vi "setUp.vi"(8 "error in (no error)":errorcluster, 11 "reference in":refnum<class "test.lvclass">) -> (0 "error out":errorcluster, 3 "reference in":refnum<class "test.lvclass">)   [LabVIEW 2011, in "test.lvclass"]
doc: "setUp runs prior to the test method during test execution. Use this method to initialize any object data required by your tests."
uses:
  test.lvclass
  test.lvclass/test.ctl
  <vilib>/addons/_JKI Toolkits/VI Tester/TestCase.llb/TestCase.lvclass
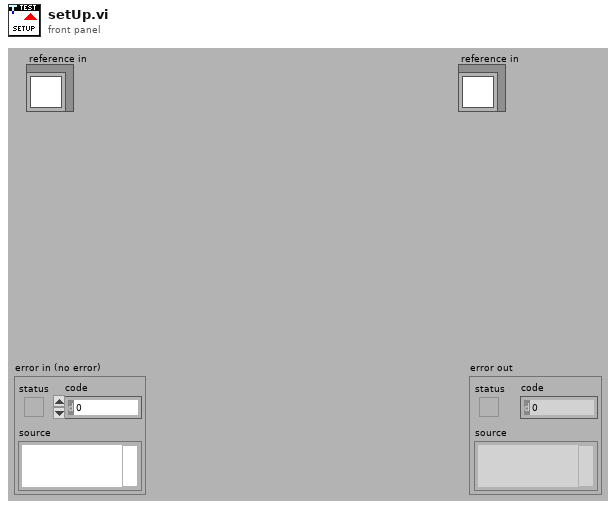
[diagram p1: front panel]
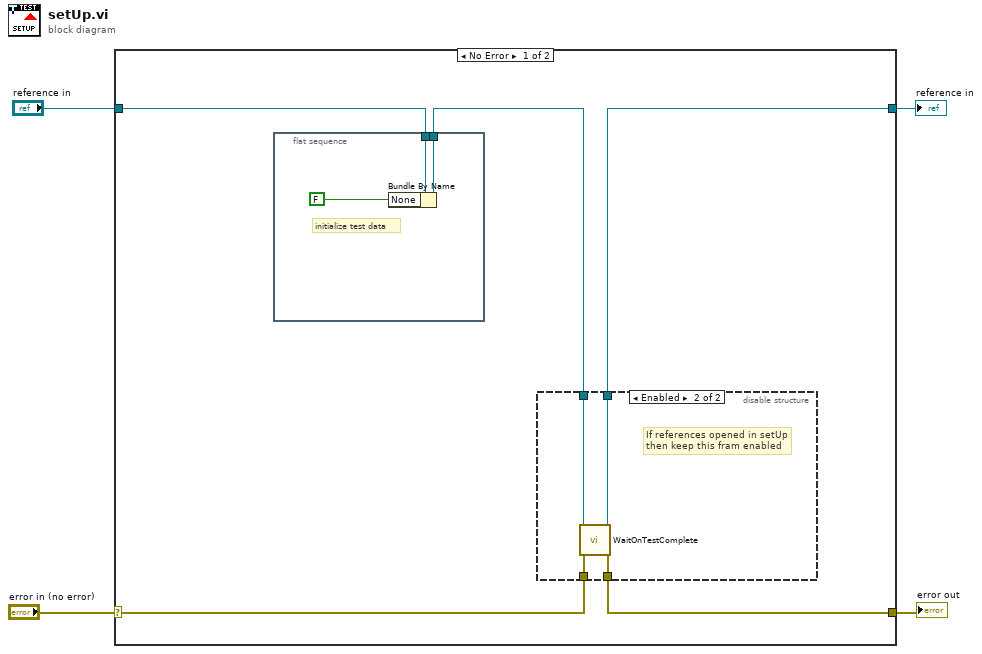
[diagram p0: block diagram]
diagram:
  n1 = case shown="No Error" "error in (no error)" {
    selector: "error in (no error)" -> [w6 w20]
    tunnel: [w5 w20] -> w3
    tunnel: [w7 w19] -> w1
    tunnel: "reference in" -> [w9 w19]
    frame No Error {
      n2 = flat-sequence {
        tunnel: w9 -> [w12]
        tunnel: [w10] -> w8
        frame #0 {
          # "initialize test data"
          n3 = Bundle By Name(cluster=w12, "None"=FALSE) -> (w10:refnum<class "test.lvclass">)
        }
      }
      n4 = disable-structure shown="Enabled" {
        disable-tunnel: w8 -> [w14 w18]
        disable-tunnel: [w14 w17] -> w7
        disable-tunnel: w6 -> [w13 w16]
        disable-tunnel: [w13 w15] -> w5
        frame Disabled {
          # "If no references opened by\nsetUp then enable this frame"
        }
        frame Enabled {
          # "If references opened in setUp\nthen keep this fram enabled"
          n5 = call <vilib>:"WaitOnTestComplete.vi"("error in (no error)"=w16, "TestCase in"=w18) -> ("error out"=w15:errorcluster, "TestCase out"=w17:refnum<class "test.lvclass">)  [unwired: 8 in]
        }
      }
    }
    frame Error {
    }
  }
  "error out" <- w3
  "reference in" <- w1
